vi "ULx Write (Analog 1D Wfm NChan NSamp).vi"(0 "task in":refnum<k24>, 1 "auto start":bool, 7 "data":waveform(dbl)[](array[waveform]), 9 "timeout":dbl=10.0 format="%_4g", 11 "error in":errorcluster) -> (4 "task out":refnum<k24>, 10 "number of samples written per channel":u32, 15 "error out":errorcluster)   [LabVIEW 2020]
doc: "Writes one or more waveforms to a task that contains one or more analog output channels."
uses:
  C:/Users/William/Documents/LV 2020 builds/LeaktestDAQ/Source-v33/ULx_LV.dll
  ULx_LV.dll
panel:
  # "channel"
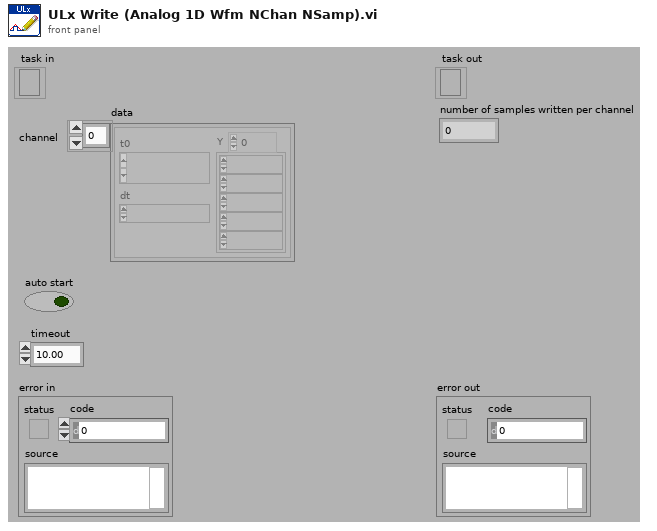
[diagram p1: front panel]
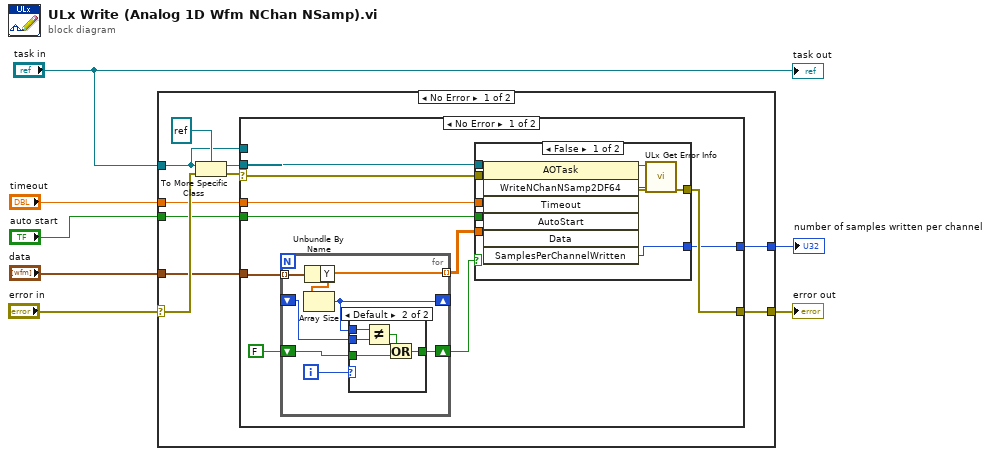
[diagram p0: block diagram]
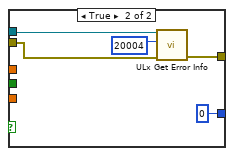
[diagram p2: hidden frame]
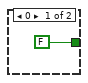
[diagram p3: hidden frame]
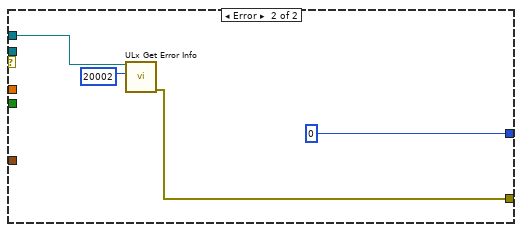
[diagram p4: hidden frame]
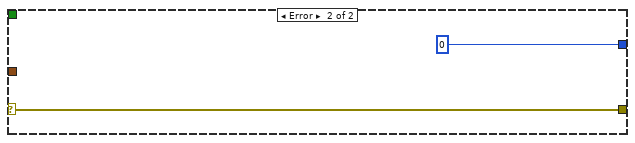
[diagram p5: hidden frame]
diagram:
  n1 = case shown="No Error" "error in" {
    selector: "error in" -> [w17 w61]
    tunnel: "task in" -> [w11 _]
    tunnel: "timeout" -> [w13 _]
    tunnel: [w12 w61] -> w5
    tunnel: "data" -> [w8 _]
    tunnel: "auto start" -> [w10 _]
    tunnel: [w9 0 ("SamplesPerChannelWritten")] -> w2
    frame No Error {
      n2 = To More Specific Class(target class=refnum<k24> refnum, reference=w11, error in=w17) -> (specific class reference=w14:refnum<k24>, error out=w15:errorcluster)
      n3 = case shown="No Error" w15 {
        selector: w15 -> [w26 _]
        tunnel: w14 -> [w27 _]
        tunnel: w13 -> [w23 _]
        tunnel: [w25 w58] -> w12
        tunnel: w11 -> [_ w57]
        tunnel: w10 -> [w22 _]
        tunnel: [w24 0 ("SamplesPerChannelWritten")] -> w9
        tunnel: w8 -> [w20 _]
        frame No Error {
          n4 = for {
            shift-right: [w48] -> _
            shift-left: _ -> [w47]
            tunnel: [w49] -> w21 mode=indexing
            tunnel: w20 -> [w46] mode=indexing
            shift-right: [w45] -> w18
            shift-left: FALSE -> [w44]
            i -> [w43]
            n5 = Unbundle By Name(w46) -> ("Y"=w49:dbl[])
            n6 = Array Size(array=w49) -> (size(s)=w48:i32)
            n7 = case shown="Default" w43 {
              tunnel: [FALSE w51] -> w45
              tunnel: w48 -> [_ w55]
              tunnel: w47 -> [_ w54]
              tunnel: w44 -> [_ w52]
              frame 0 {
              }
              frame Default {
                n8 = Not Equal?(x=w55, y=w54) -> (x != y?=w53:bool)
                n9 = Or(x=w53, y=w52) -> (x .or. y?=w51:bool)
              }
            }
          }
          n10 = case shown="False" w18 {
            tunnel: w27 -> [w37 w39]
            tunnel: w26 -> [w36 w38]
            tunnel: [w33 w42] -> w25
            tunnel: [w31 u32 0 ("SamplesPerChannelWritten")] -> w24
            tunnel: w23 -> [w30 _]
            tunnel: w22 -> [w29 _]
            tunnel: w21 -> [w28 _]
            frame False {
              n11 = invoke class="AOTask" method="WriteNChanNSamp2DF64"(reference=w37, error in=w36, "Timeout"=w30, "AutoStart"=w29, "Data"=w28) -> (reference out=w34:refnum<k24>, error out=w35:errorcluster, "WriteNChanNSamp2DF64"=w32:i32, "SamplesPerChannelWritten"=w31:u32)  [unwired: 2 in, 3 out]
              n12 = call "ULx Get Error Info.vi"("error in"=w35, "ErrorCode"=w32, "task in"=w34) -> ("error out"=w33:errorcluster)  [unwired: 8 in]
            }
            frame True {
              n13 = call "ULx Get Error Info.vi"("error in"=w38, "ErrorCode"=20004, "task in"=w39) -> ("error out"=w42:errorcluster)  [unwired: 8 in]
            }
          }
        }
        frame Error {
          n14 = call "ULx Get Error Info.vi"("ErrorCode"=20002, "task in"=w57) -> ("error out"=w58:errorcluster)  [unwired: 9 in]
        }
      }
    }
    frame Error {
    }
  }
  "error out" <- w5
  "number of samples written per channel" <- w2
  "task out" <- "task in"
